vi "Teleop.vi"(10 "Match Info":T1={"Autonomous Elapsed Seconds"=0.0, "TeleOp Elapsed Seconds"=0.0, "Disabled Elapsed Seconds"=0.0, "Visited Autonomous"=FALSE, "Visited TeleOp"=FALSE, "Visited Disabled"=FALSE, "Autonomous Settings"={"Autonomous Style"=enum."Independent", "VI Refnum"=refnum}}, 11 "Call Context":T2) -> ()   [LabVIEW 2016]
doc: "This VI is called for each TeleOp packet received from the DS where the robot is not disabled. It is often used to read from the joysticks and update I/O or to update setpoints for timed control loops. It should complete and return within 20 milliseconds or it may miss DS packets."
uses:
  <vilib>/Rock Robotics/WPI/Solenoid/WPI_SolenoidValue.ctl
  <vilib>/Rock Robotics/WPI/Solenoid/WPI_SolenoidSetEnum.vi
  <vilib>/Rock Robotics/WPI/DriverStation/WPI_DriverStationMatch Info.ctl
  <vilib>/Rock Robotics/WPI/DriverStation/WPI_DriverStationDerivedRobotMode.ctl
panel:
  in  "Range":dbl=25.0 format="%#_13g"
  out "Encoder Position R":dbl
  out "Encoder Position L":dbl
  out "Gyro Angle":dbl format="%#_13g"
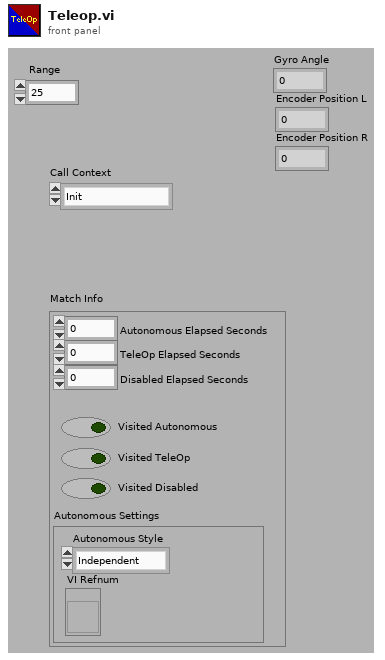
[diagram p1: front panel]
types:
  T1 = typedef "WPI_DriverStationMatch Info.ctl" = cluster{"Autonomous Elapsed Seconds":dbl, "TeleOp Elapsed Seconds":dbl, "Disabled Elapsed Seconds":dbl, "Visited Autonomous":bool, "Visited TeleOp":bool, "Visited Disabled":bool, "Autonomous Settings":cluster{"Autonomous Style":enum16{"Iterative", "Independent"}, "VI Refnum":refnum<vi>}}
  T2 = typedef "WPI_DriverStationDerivedRobotMode.ctl" = enum16{"Init", "Execute", "Stop"}
  T3 = typedef "WPI_SolenoidValue.ctl" = enum16{"Off", "On", "Forward", "Reverse"}
  T4 = typedef "WPI_GyroDevRef.ctl" = cluster{"DevStatus":errorcluster, "Analog Channel":T5, "Offset":dbl, "Gain (VoltsPerDegree/Second)":dbl, "Gyro Type":enum16{"Analog", "XRS450"}, "Handle":i32, "SPI Bus":T6, "Device Found":bool, "Sample Rate":dbl, "Calibrate On Open":bool}
  T5 = typedef "FPGA_AIChannel.ctl" = enum8{"AI 0", "AI 1", "AI 2", "AI 3", "AI MXP 0", "AI MXP 1", "AI MXP 2", "AI MXP 3", "Invalid"}
  T6 = typedef "spi_bus.ctl" = enum16{"SPI On-Board, CS0", "SPI On-Board, CS1", "SPI On-Board, CS2", "SPI On-Board, CS3", "SPI MXP", "Invalid"}
  T7 = typedef "WPI_JoystickDevRef.ctl" = cluster{"Device":T8}
  T8 = typedef "WPI_JoystickDeviceEnum.ctl" = enum16{"USB 0", "USB 1", "USB 2", "USB 3", "USB 4", "USB 5"}
  T9 = typedef "WPI_MotorControlDeviceRef.ctl" = cluster{"DeviceStatus":errorcluster, "Type":T10, "PWM":cluster{"PWM Channel":T11, "DeadBand":T12}, "CAN":cluster{"Device Number":u8, "SetOutput VI Ref":variant, "GetOutput VI Ref":variant, "Enable VI Ref":variant, "Disable VI Ref":variant, "Data":variant}, "Invert":bool}
  T10 = typedef "WPI_MotorControlType.ctl" = enum16{"PWM", "CAN"}
  T11 = typedef "FPGA_DIOPWMChannel.ctl" = enum8{"PWM 0", "PWM 1", "PWM 2", "PWM 3", "PWM 4", "PWM 5", "PWM 6", "PWM 7", "PWM 8", "PWM 9", "PWM MXP 0", "PWM MXP 1", "PWM MXP 2", "PWM MXP 3", "PWM MXP 4", "PWM MXP 5", "PWM MXP 6", "PWM MXP 7", "PWM MXP 8", "PWM MXP 9", "Invalid"}
  T12 = typedef "WPI_PWMDeadband.ctl" = cluster{"Name":string, "maxPositivePwm":i32, "minPositivePwm":i32, "centerPwm":i32, "maxNegativePwm":i32, "minNegativePwm":i32, "angularRange":u16}
  T13 = typedef "WPI_CANTalonSRX_GlobalStatus.ctl" = cluster{"Applied Throttle":dbl, "Module Enabled":bool, "CAN Error":errorcluster, "Closed Loop Error":dbl, "Forward Limit Switch Closed":bool, "Reverse Limit Switch Closed":bool, "Sensor Position":dbl, "Sensor Velocity":dbl, "Current":dbl, "Sticky Fault - Over Temp":bool, "Sticky Fault - Under Voltage":bool, "Sticky Fault - Forward Limit":bool, "Sticky Fault - Reverse Limit":bool, "Sticky Fault - Forward Soft Limit":bool, "Sticky Fault - Reverse Soft Limit":bool, "Brake is Enabled":bool, "Encoder Position":dbl, "Encoder Velocity":dbl, "Encoder Index Count":dbl, "Encoder A Pin State":bool, "Encoder B Pin State":bool, "Encoder Index Pin State":bool, "Analog In":dbl, "Analog In Velocity":dbl, "Temperature (C)":dbl, "Battery Voltage":dbl, "Control 5 Is Supported":bool, "Current Profile Slot Select":dbl, "Pos Div 8":bool, "Vel Div 4":bool, "Pulse Width Position":i32, "Pulse Width Velocity":i32, "Pulse Width Rise To Rise (us)":i32, "Pulse Width Rise To Fall (us)":i32, "Mot Prof Active Is Under Run":bool, "Mot Prof Active Has Under Run":bool, "Mot Prof Active Is Last":bool, "Mot Prof Active Velocity Only":bool, "Mot Prof Active Is Valid":bool, "Mot Prof Buffer Is Full":bool, "Mot Prof Active Profile Slot Select":i32, "Mot Prof NextID":i32, "Mot Prof Count":i32, "Mot Prof Active Velocity":dbl, "Mot Prof Active Position":dbl, "Mot Prof Output Enable":i32}
  T14 = typedef "WPI_SolenoidDevRef.ctl" = cluster{"DevStatus":errorcluster, "Pneumatics Control Module":u8, "Forward Solenoid Channel":T15, "Reverse Solenoid Channel":T15}
  T15 = typedef "WPI_SolenoidChannel.ctl" = enum8{"Solenoid 0", "Solenoid 1", "Solenoid 2", "Solenoid 3", "Solenoid 4", "Solenoid 5", "Solenoid 6", "Solenoid 7", "Invalid"}
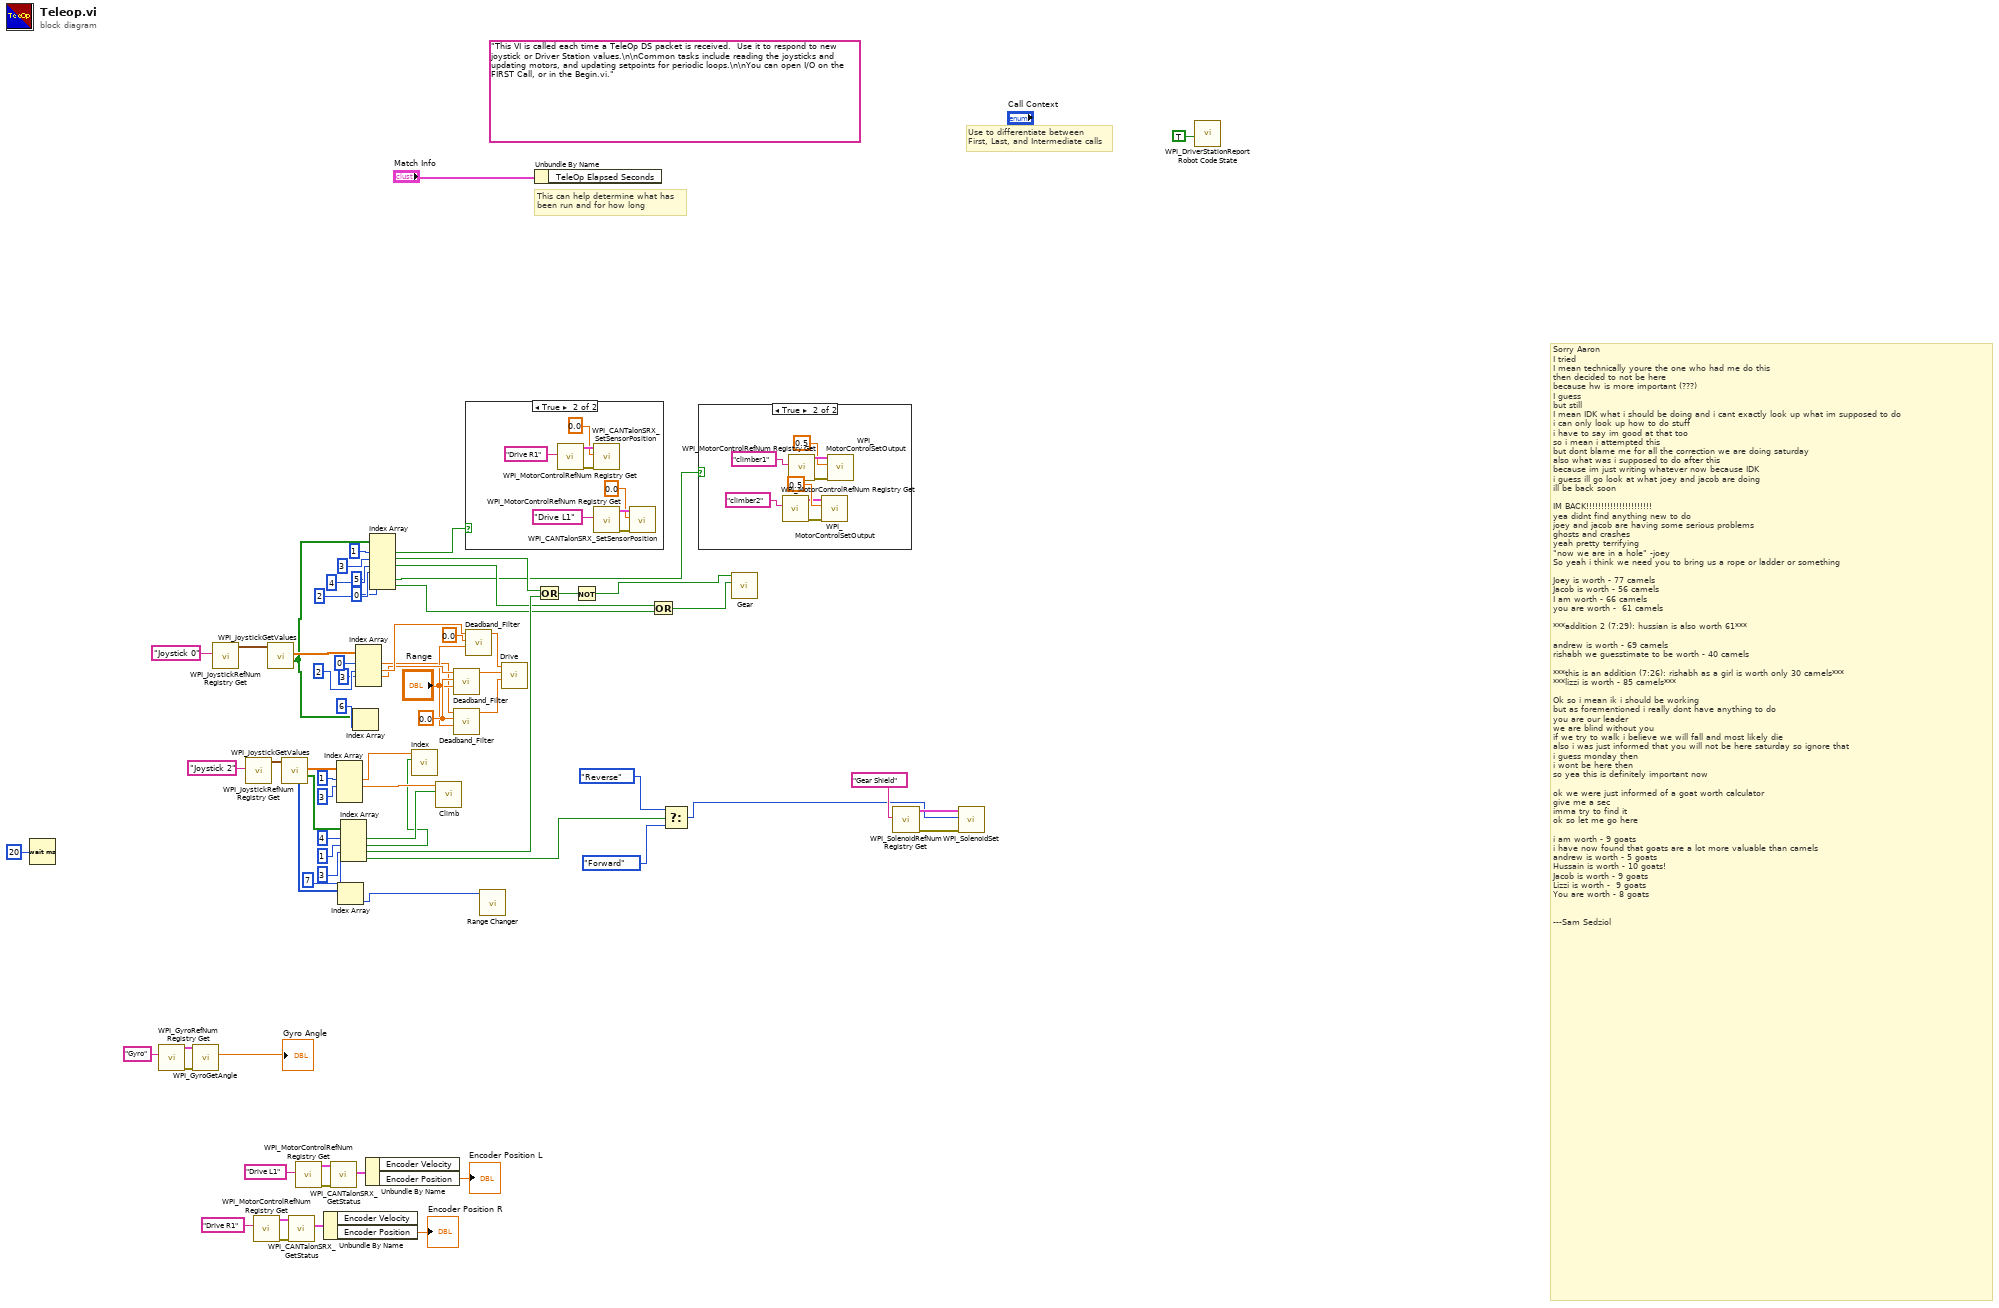
[diagram p0: block diagram]
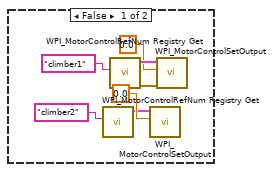
[diagram p2: hidden frame]
diagram:
  w7 = 0.0 ("Target")
  (unwired) "This VI is called each time a TeleOp DS packet is received.  Use it to respond to new joystick or Driver Station values.\n\nCommon tasks include reading the joysticks and updating motors, and updating setpoints for periodic loops.\n\nYou can open I/O on the FIRST Call, or in the Begin.vi."
  # "Sorry Aaron\nI tried\nI mean technically youre the one who had me do this\nthen decided to not be here\nbecause hw is more important (???)\nI guess\nbut still\nI mean IDK what i should be doing and i cant exactly look up what im supposed to do\ni can only look up how to do stuff\ni have to say im good at that too\nso i mean i attempted this\nbut dont blame me for all the correction we are doing saturday\nalso what was i supposed to do after this\nbecause im just writing whatever now because IDK\ni guess ill go look at what joey and jacob are doing\nill be back soon\n\nIM BACK!!!!!!!!!!!!!!!!!!!!!!\nyea didnt find anything new to do\njoey and jacob are having some serious problems\nghosts and crashes\nyeah pretty terrifying\n\"now we are in a hole\" -joey\nSo yeah i think we need you to bring us a rope or ladder or something\n\nJoey is worth - 77 camels\nJacob is worth - 56 camels\nI am worth - 66 camels\nyou are worth -  61 camels \n\n***addition 2 (7:29): hussian is also worth 61***\n\nandrew is worth - 69 camels\nrishabh we guesstimate to be worth - 40 camels\n\n***this is an addition (7:26): rishabh as a girl is worth only 30 camels***\n***lizzi is worth - 85 camels***\n\nOk so i mean ik i should be working\nbut as forementioned i really dont have anything to do\nyou are our leader\nwe are blind without you\nif we try to walk i believe we will fall and most likely die\nalso i was just informed that you will not be here saturday so ignore that\ni guess monday then\ni wont be here then\nso yea this is definitely important now\n\nok we were just informed of a goat worth calculator\ngive me a sec \nimma try to find it\nok so let me go here\n\ni am worth - 9 goats\ni have now found that goats are a lot more valuable than camels\nandrew is worth - 5 goats\nHussain is worth - 10 goats! \nJacob is worth - 9 goats\nLizzi is worth -  9 goats\nYou are worth - 8 goats\n\n\n---Sam Sedziol"
  # "Use to differentiate between\nFirst, Last, and Intermediate calls"
  # "This can help determine what has\nbeen run and for how long"
  n1 = Wait (ms)(milliseconds to wait=u32 20) -> ()  [unwired: 1 out]
  n2 = call <vilib>:"WPI_GyroRefNum Registry Get.vi"("refnum name"="Gyro") -> ("error out"=w54:errorcluster, "GyroDevRef"=w53:T4)  [unwired: 9 in]
  n3 = call <vilib>:"WPI_GyroGetAngle.vi"("error in"=w54, "GyroDevRef"=w53) -> ("Angle"=→"Gyro Angle":dbl)  [unwired: 5 in, 4 out]
  n4 = call <vilib>:"WPI_JoystickRefNum Registry Get.vi"("refnum name"="Joystick 0") -> ("JoystickDevRef"=w60:T7)  [unwired: 1 in, 9 out]
  n5 = call <vilib>:"WPI_JoystickRefNum Registry Get.vi"("refnum name"="Joystick 2") -> ("JoystickDevRef"=w67:T7)  [unwired: 1 in, 9 out]
  n6 = call <vilib>:"WPI_MotorControlRefNum Registry Get.vi"("refnum name"="Drive R1") -> ("error out"=w48:errorcluster, "MotorControlDevRef"=w49:T9)  [unwired: 9 in]
  n7 = call <vilib>:"WPI_JoystickGetValues.vi"("JoystickDevRef"=w60) -> ("Buttons"=w14:bool[], "Axes"=w69:dbl[])  [unwired: 6 in, 3 out]
  n8 = call <vilib>:"WPI_JoystickGetValues.vi"("JoystickDevRef"=w67) -> ("Buttons"=w65:bool[], "Axes"=w66:dbl[], "POVs"=w27:i16[])  [unwired: 6 in, 2 out]
  n9 = call <vilib>:"WPI_CANTalonSRX_GetStatus.vi"("error in (no error)"=w48, "CAN Talon SRX Ref"=w49) -> ("Talon SRX Status"=w46:T13)  [unwired: 7 in, 2 out]
  n10 = call <vilib>:"WPI_MotorControlRefNum Registry Get.vi"("refnum name"="Drive L1") -> ("error out"=w45:errorcluster, "MotorControlDevRef"=w50:T9)  [unwired: 9 in]
  n11 = Unbundle By Name(w46) -> ("Encoder Position"=→"Encoder Position R":dbl)  [unwired: 1 out]
  n12 = call <vilib>:"WPI_CANTalonSRX_GetStatus.vi"("error in (no error)"=w45, "CAN Talon SRX Ref"=w50) -> ("Talon SRX Status"=w47:T13)  [unwired: 7 in, 2 out]
  n13 = Index Array(array=w66, index #1=1 ("index"), index #2=3 ("index")) -> (element #1=w40:dbl, element #2=w61:dbl)  [unwired: 2 in, 2 out]
  n14 = Index Array(array=w27) -> (element=w26:i16)  [unwired: 1 in]
  n15 = Index Array(array=w65, index #1=4 ("index"), index #2=1 ("index"), index #3=3 ("index"), index #4=7) -> (element #1=w36:bool, element #2=w17:bool, element #3=w37:bool, element #4=w20:bool)
  n16 = Index Array(array=w14, index=6) -> ()  [unwired: 1 out]
  n17 = Index Array(array=w69, index #1=0 ("index"), index #2=2 ("index"), index #3=3 ("index")) -> (element #1=w3:dbl, element #2=w13:dbl, element #3=w6:dbl)  [unwired: 1 in, 1 out]
  n18 = Unbundle By Name(w47) -> ("Encoder Position"=→"Encoder Position L":dbl)  [unwired: 1 out]
  n19 = Index Array(array=w14, index #1=1 ("index"), index #2=3 ("index"), index #3=4 ("index"), index #4=2 ("index"), index #5=5 ("index"), index #6=0 ("index")) -> (element #1=w63:bool, element #2=w32:bool, element #3=w31:bool, element #5=w15:bool, element #6=w1:bool)  [unwired: 1 out]
  n20 = call "Index.vi"("Shoot"=w17, "Output"=w40) -> ()  [unwired: 10 in]
  n21 = call "Climb.vi"("Backwards?"=w36, "Effort"=w61) -> ()  [unwired: 10 in]
  n22 = call "Deadband_Filter.vi"("Range"="Range", "Target"=w7, "Joystick Input"=w6) -> ("Output"=w4:dbl)  [unwired: 8 in]
  n23 = call "Deadband_Filter.vi"("Range"="Range", "Target"=w7, "Joystick Input"=w3) -> ("Output"=w9:dbl)  [unwired: 8 in]
  n24 = case shown="True" w63 {
    frame False {
    }
    frame True {
      n25 = call <vilib>:"WPI_MotorControlRefNum Registry Get.vi"("refnum name"="Drive R1") -> ("error out"=w75:errorcluster, "MotorControlDevRef"=w74:T9)  [unwired: 9 in]
      n26 = call <vilib>:"WPI_CANTalonSRX_SetSensorPosition.vi"("error in (no error)"=w75, "New Sensor Position"=0.0, "CAN Talon SRX Ref"=w74) -> ()  [unwired: 7 in, 2 out]
      n27 = call <vilib>:"WPI_MotorControlRefNum Registry Get.vi"("refnum name"="Drive L1") -> ("error out"=w77:errorcluster, "MotorControlDevRef"=w78:T9)  [unwired: 9 in]
      n28 = call <vilib>:"WPI_CANTalonSRX_SetSensorPosition.vi"("error in (no error)"=w77, "New Sensor Position"=0.0, "CAN Talon SRX Ref"=w78) -> ()  [unwired: 7 in, 2 out]
    }
  }
  n29 = call "Deadband_Filter.vi"("Range"="Range", "Target"=0.0, "Joystick Input"=w13) -> ("Output"=w8:dbl)  [unwired: 8 in]
  n30 = call "Range Changer.vi"("POV"=w26) -> ()  [unwired: 10 in, 1 out]
  n31 = call "Drive.vi"("Joystick 1"=w9, "RT"=w4, "LT"=w8) -> ()  [unwired: 9 in]
  n32 = Unbundle By Name("Match Info") -> ()  [unwired: 1 out]
  n33 = Or(x=w32, y=w37) -> (x .or. y?=w55:bool)
  n34 = Not(x=w55) -> (.not. x?=w30:bool)
  n35 = Or(x=w31, y=w1) -> (x .or. y?=w29:bool)
  n36 = Select(t=WPI_SolenoidValue."Reverse" ("Value"), s=w20, f=WPI_SolenoidValue."Forward" ("Value")) -> (s? t:f=w18:T3)
  n37 = case shown="True" w15 {
    frame False {
      n38 = call <vilib>:"WPI_MotorControlRefNum Registry Get.vi"("refnum name"="climber2") -> ("MotorControlDevRef"=w82:T9)  [unwired: 9 in, 1 out]
      n39 = call <vilib>:"WPI_MotorControlRefNum Registry Get.vi"("refnum name"="climber1") -> ("error out"=w86:errorcluster, "MotorControlDevRef"=w85:T9)  [unwired: 9 in]
      n40 = call <vilib>:"WPI_MotorControlSetOutput.vi"("Output"=0.0, "MotorControlDevRef"=w82) -> ()  [unwired: 7 in, 3 out]
      n41 = call <vilib>:"WPI_MotorControlSetOutput.vi"("error in (no error)"=w86, "Output"=0.0, "MotorControlDevRef"=w85) -> ()  [unwired: 6 in, 3 out]
    }
    frame True {
      n42 = call <vilib>:"WPI_MotorControlRefNum Registry Get.vi"("refnum name"="climber2") -> ("error out"=w89:errorcluster, "MotorControlDevRef"=w90:T9)  [unwired: 9 in]
      n43 = call <vilib>:"WPI_MotorControlRefNum Registry Get.vi"("refnum name"="climber1") -> ("error out"=w94:errorcluster, "MotorControlDevRef"=w93:T9)  [unwired: 9 in]
      n44 = call <vilib>:"WPI_MotorControlSetOutput.vi"("error in (no error)"=w89, "Output"=0.5, "MotorControlDevRef"=w90) -> ()  [unwired: 6 in, 3 out]
      n45 = call <vilib>:"WPI_MotorControlSetOutput.vi"("error in (no error)"=w94, "Output"=0.5, "MotorControlDevRef"=w93) -> ()  [unwired: 6 in, 3 out]
    }
  }
  n46 = call "Gear.vi"("Gear0?"=w29, "Gear1?"=w30) -> ()  [unwired: 10 in]
  n47 = call <vilib>:"WPI_SolenoidRefNum Registry Get.vi"("refnum name"="Gear Shield") -> ("error out"=w23:errorcluster, "SolenoidDevRef"=w22:T14)  [unwired: 9 in]
  n48 = call-poly <vilib>:"WPI_SolenoidSet.vi"("error in (no error)"=w23, "Value"=w18, "SolenoidDevRef"=w22) -> ()  [unwired: 7 in, 2 out]
  n49 = call <vilib>:"WPI_DriverStationReport Robot Code State.vi"("TeleOp"=TRUE ("Autonomous")) -> ()  [unwired: 10 in, 1 out]
